vi "Input the Password.vi"() -> (0 "数字":dbl format="%#.10f", 1 "字符串":string, 2 "数据是否有效":bool=TRUE)   [LabVIEW 2017]
doc: "模拟键盘"
uses:
  MSVCRT.DLL
panel:
  in  "确定":bool
  in  "后退":bool
  in  "取消":bool
  in  "6":bool
  in  "3":bool
  in  "9":bool
  in  "5":bool
  in  "2":bool
  in  "8":bool
  out "小数点可用s":bool=TRUE
  in  "0":bool
  in  "4":bool
  in  "1":bool
  in  "7":bool
  # "Password"
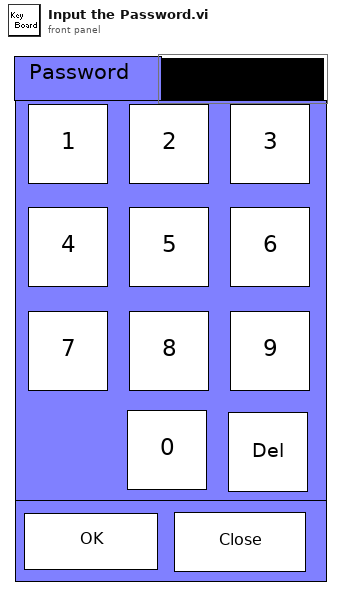
[diagram p1: front panel]
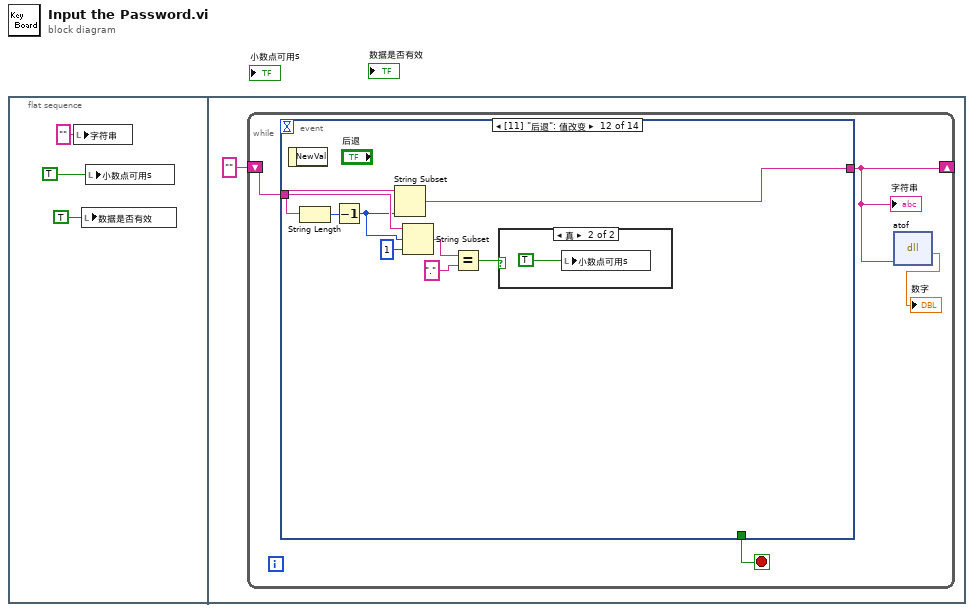
[diagram p0: block diagram]
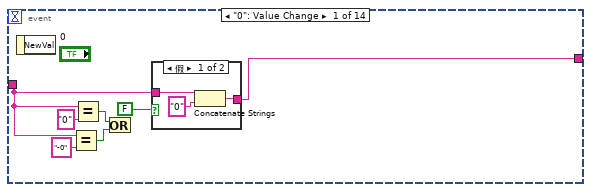
[diagram p2: hidden frame]
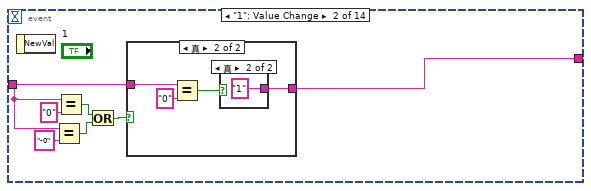
[diagram p4: hidden frame]
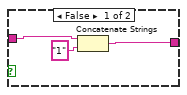
[diagram p5: hidden frame]
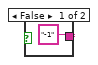
[diagram p6: hidden frame]
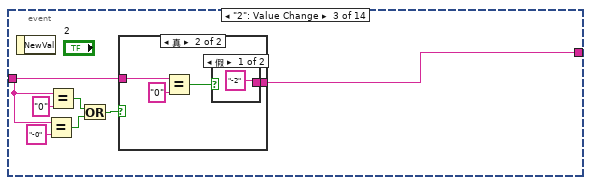
[diagram p7: hidden frame]
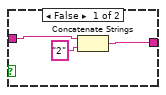
[diagram p8: hidden frame]
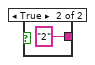
[diagram p9: hidden frame]
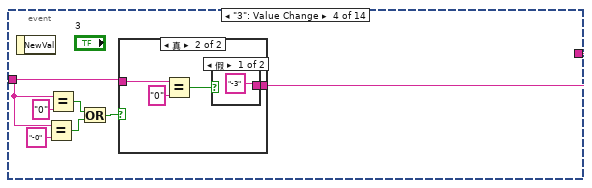
[diagram p10: hidden frame]
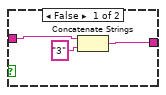
[diagram p11: hidden frame]
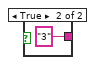
[diagram p12: hidden frame]
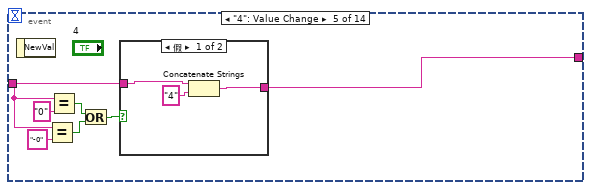
[diagram p13: hidden frame]
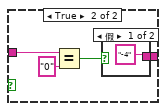
[diagram p14: hidden frame]
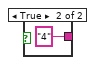
[diagram p15: hidden frame]
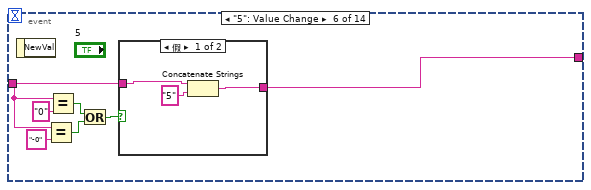
[diagram p16: hidden frame]
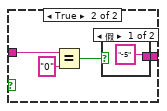
[diagram p17: hidden frame]
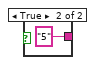
[diagram p18: hidden frame]
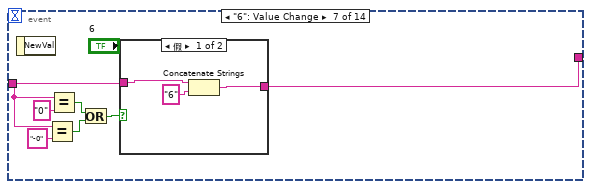
[diagram p19: hidden frame]
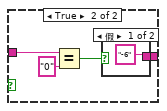
[diagram p20: hidden frame]
diagram:
  n1 = flat-sequence {
    frame #0 {
      n2 = local write "字符串"("" ("字符串")) -> ()
      n3 = local write "数据是否有效"(TRUE ("数据是否有效")) -> ()
      n4 = local write "小数点可用s"(TRUE ("第一次使用小数点")) -> ()
    }
    frame #1 {
      n5 = while {
        shift-right: [w6] -> _
        shift-left: "" ("字符串") -> [w7]
        stop <- w8 stop-if-true
        n6 = event shown="[11] \"后退\": 值改变" {
          selector: _ -> [_ _ _ _ _ _ _ _ _ _ _ _ _ _]
          dyn-events: _ -> [_ _ _ _ _ _ _ _ _ _ _ _ _ _]
          timeout: _ -> [_ _ _ _ _ _ _ _ _ _ _ _ _ _]
          tunnel: [_ _ _ _ _ _ _ _ _ _ "确定" _ w175 TRUE ("NewVal")] -> w8
          tunnel: w7 -> [w11 w21 w37 w53 w69 w85 w101 w117 w133 w149 w164 w171 _ _]
          tunnel: [w10 w20 w36 w52 w68 w84 w100 w116 w132 w148 w164 w172 _ _] -> w6
          event "0": Value Change {
            n7 = event-data() -> ()  [unwired: 1 in, 1 out]
            n8 = Equal?(x=w11, y="-0") -> (x = y?=w13:bool)
            n9 = Equal?(x=w11, y="0") -> (x = y?=w12:bool)
            n10 = Or(x=w12, y=w13) -> ()  [unwired: 1 out]
            n11 = case shown="假" FALSE {
              tunnel: w11 -> [w18 w19]
              tunnel: [w17 w19] -> w10
              frame False {
                n12 = Concatenate Strings(w18, "0" ("字符串")) -> (w17:string)
              }
              frame True {
              }
            }
          }
          event "1": Value Change {
            n13 = event-data() -> ()  [unwired: 1 in, 1 out]
            n14 = Equal?(x=w21, y="-0") -> (x = y?=w24:bool)
            n15 = Equal?(x=w21, y="0") -> (x = y?=w23:bool)
            n16 = Or(x=w23, y=w24) -> (x .or. y?=w22:bool)
            n17 = case shown="真" w22 {
              tunnel: w21 -> [w28 w32]
              tunnel: [w27 w30] -> w20
              frame False {
                n18 = Concatenate Strings(w28, "1" ("字符串")) -> (w27:string)
              }
              frame True {
                n19 = Equal?(x=w32, y="0") -> (x = y?=w31:bool)
                n20 = case shown="真" w31 {
                  tunnel: ["-1" ("y") "1" ("y")] -> w30
                  frame False {
                  }
                  frame True {
                  }
                }
              }
            }
          }
          event "2": Value Change {
            n21 = event-data() -> ()  [unwired: 1 in, 1 out]
            n22 = Equal?(x=w37, y="-0") -> (x = y?=w40:bool)
            n23 = Equal?(x=w37, y="0") -> (x = y?=w39:bool)
            n24 = Or(x=w39, y=w40) -> (x .or. y?=w38:bool)
            n25 = case shown="真" w38 {
              tunnel: w37 -> [w44 w48]
              tunnel: [w43 w46] -> w36
              frame False {
                n26 = Concatenate Strings(w44, "2" ("字符串")) -> (w43:string)
              }
              frame True {
                n27 = Equal?(x=w48, y="0") -> (x = y?=w47:bool)
                n28 = case shown="假" w47 {
                  tunnel: ["-2" ("y") "2" ("y")] -> w46
                  frame False {
                  }
                  frame True {
                  }
                }
              }
            }
          }
          event "3": Value Change {
            n29 = event-data() -> ()  [unwired: 1 in, 1 out]
            n30 = Equal?(x=w53, y="-0") -> (x = y?=w56:bool)
            n31 = Equal?(x=w53, y="0") -> (x = y?=w55:bool)
            n32 = Or(x=w55, y=w56) -> (x .or. y?=w54:bool)
            n33 = case shown="真" w54 {
              tunnel: w53 -> [w60 w64]
              tunnel: [w59 w62] -> w52
              frame False {
                n34 = Concatenate Strings(w60, "3" ("字符串")) -> (w59:string)
              }
              frame True {
                n35 = Equal?(x=w64, y="0") -> (x = y?=w63:bool)
                n36 = case shown="假" w63 {
                  tunnel: ["-3" ("y") "3" ("y")] -> w62
                  frame False {
                  }
                  frame True {
                  }
                }
              }
            }
          }
          event "4": Value Change {
            n37 = event-data() -> ()  [unwired: 1 in, 1 out]
            n38 = Equal?(x=w69, y="-0") -> (x = y?=w72:bool)
            n39 = Equal?(x=w69, y="0") -> (x = y?=w71:bool)
            n40 = Or(x=w71, y=w72) -> (x .or. y?=w70:bool)
            n41 = case shown="假" w70 {
              tunnel: w69 -> [w76 w80]
              tunnel: [w75 w78] -> w68
              frame False {
                n42 = Concatenate Strings(w76, "4" ("字符串")) -> (w75:string)
              }
              frame True {
                n43 = Equal?(x=w80, y="0") -> (x = y?=w79:bool)
                n44 = case shown="假" w79 {
                  tunnel: ["-4" ("y") "4" ("y")] -> w78
                  frame False {
                  }
                  frame True {
                  }
                }
              }
            }
          }
          event "5": Value Change {
            n45 = event-data() -> ()  [unwired: 1 in, 1 out]
            n46 = Equal?(x=w85, y="-0") -> (x = y?=w88:bool)
            n47 = Equal?(x=w85, y="0") -> (x = y?=w87:bool)
            n48 = Or(x=w87, y=w88) -> (x .or. y?=w86:bool)
            n49 = case shown="假" w86 {
              tunnel: w85 -> [w92 w96]
              tunnel: [w91 w94] -> w84
              frame False {
                n50 = Concatenate Strings(w92, "5" ("字符串")) -> (w91:string)
              }
              frame True {
                n51 = Equal?(x=w96, y="0") -> (x = y?=w95:bool)
                n52 = case shown="假" w95 {
                  tunnel: ["-5" ("y") "5" ("y")] -> w94
                  frame False {
                  }
                  frame True {
                  }
                }
              }
            }
          }
          event "6": Value Change {
            n53 = event-data() -> ()  [unwired: 1 in, 1 out]
            n54 = Equal?(x=w101, y="-0") -> (x = y?=w104:bool)
            n55 = Equal?(x=w101, y="0") -> (x = y?=w103:bool)
            n56 = Or(x=w103, y=w104) -> (x .or. y?=w102:bool)
            n57 = case shown="假" w102 {
              tunnel: w101 -> [w108 w112]
              tunnel: [w107 w110] -> w100
              frame False {
                n58 = Concatenate Strings(w108, "6" ("字符串")) -> (w107:string)
              }
              frame True {
                n59 = Equal?(x=w112, y="0") -> (x = y?=w111:bool)
                n60 = case shown="假" w111 {
                  tunnel: ["-6" ("y") "6" ("y")] -> w110
                  frame False {
                  }
                  frame True {
                  }
                }
              }
            }
          }
          event "7": Value Change {
            n61 = event-data() -> ()  [unwired: 1 in, 1 out]
            n62 = Equal?(x=w117, y="-0") -> (x = y?=w120:bool)
            n63 = Equal?(x=w117, y="0") -> (x = y?=w119:bool)
            n64 = Or(x=w119, y=w120) -> (x .or. y?=w118:bool)
            n65 = case shown="假" w118 {
              tunnel: w117 -> [w124 w128]
              tunnel: [w123 w126] -> w116
              frame False {
                n66 = Concatenate Strings(w124, "7" ("字符串")) -> (w123:string)
              }
              frame True {
                n67 = Equal?(x=w128, y="0") -> (x = y?=w127:bool)
                n68 = case shown="假" w127 {
                  tunnel: ["-7" ("y") "7" ("y")] -> w126
                  frame False {
                  }
                  frame True {
                  }
                }
              }
            }
          }
          event "8": Value Change {
            n69 = event-data() -> ()  [unwired: 1 in, 1 out]
            n70 = Equal?(x=w133, y="-0") -> (x = y?=w136:bool)
            n71 = Equal?(x=w133, y="0") -> (x = y?=w135:bool)
            n72 = Or(x=w135, y=w136) -> (x .or. y?=w134:bool)
            n73 = case shown="假" w134 {
              tunnel: w133 -> [w140 w144]
              tunnel: [w139 w142] -> w132
              frame False {
                n74 = Concatenate Strings(w140, "8" ("字符串")) -> (w139:string)
              }
              frame True {
                n75 = Equal?(x=w144, y="0") -> (x = y?=w143:bool)
                n76 = case shown="假" w143 {
                  tunnel: ["-8" ("y") "8" ("y")] -> w142
                  frame False {
                  }
                  frame True {
                  }
                }
              }
            }
          }
          event "9": Value Change {
            n77 = event-data() -> ()  [unwired: 1 in, 1 out]
            n78 = Equal?(x=w149, y="-0") -> (x = y?=w152:bool)
            n79 = Equal?(x=w149, y="0") -> (x = y?=w151:bool)
            n80 = Or(x=w151, y=w152) -> (x .or. y?=w150:bool)
            n81 = case shown="假" w150 {
              tunnel: w149 -> [w156 w160]
              tunnel: [w155 w158] -> w148
              frame False {
                n82 = Concatenate Strings(w156, "9" ("字符串")) -> (w155:string)
              }
              frame True {
                n83 = Equal?(x=w160, y="0") -> (x = y?=w159:bool)
                n84 = case shown="假" w159 {
                  tunnel: ["-9" ("y") "9" ("y")] -> w158
                  frame False {
                  }
                  frame True {
                  }
                }
              }
            }
          }
          event "确定": Value Change {
            n85 = event-data() -> ()  [unwired: 1 in, 1 out]
          }
          event "后退": Value Change {
            n86 = event-data() -> ()  [unwired: 1 in, 1 out]
            n87 = String Length(string=w171) -> (length=w173:i32)
            n88 = Decrement(x=w173) -> (x-1=w170:i32)
            n89 = String Subset(string=w171, length (rest)=w170) -> (substring=w172:string)  [unwired: 1 in]
            n90 = String Subset(string=w171, offset (0)=w170, length (rest)=1 ("长度（剩余）")) -> (substring=w168:string)
            n91 = Equal?(x=w168, y=".") -> (x = y?=w166:bool)
            n92 = case shown="真" w166 {
              frame False {
              }
              frame True {
                n93 = local write "小数点可用s"(TRUE ("第一次使用小数点")) -> ()
              }
            }
          }
          event "取消": Value Change {
            n94 = event-data() -> ("NewVal"=w175:bool)  [unwired: 1 in]
            n95 = local write "数据是否有效"(FALSE ("数据是否有效")) -> ()
          }
          event Panel Close? {
            n96 = event-data() -> ()  [unwired: 1 in, 1 out]
            n97 = local write "数据是否有效"(FALSE ("数据是否有效")) -> ()
            n98 = event-data() -> ()  [unwired: 2 in, 1 out]
          }
        }
        "字符串" <- w6
        n99 = dll-call lib="MSVCRT.DLL" fn="atof"("参数1"=w6) -> ("返回类型"=→"数字":dbl)  [unwired: 4 in, 2 out]
      }
    }
  }
